vi "generate channels from bitfile registers.vi"(8 "error in":errorcluster, 11 "bitfilefile path":path) -> (0 "error out":errorcluster, 2 "not supported channels":refnum<class "TBM channel.lvclass">[](array[class]), 3 "channels":refnum<class "TBM channel.lvclass">[](array[class]))   [LabVIEW 2014, in "io configuration.lvclass"]
uses:
  io configuration.lvclass
  <vilib>/NI/Tag Bus Module Framework/channel/channel classification.ctl
  <vilib>/NI/Tag Bus Module Framework/channel/TBM channel.lvclass
  <vilib>/NI/Tag Bus/tag/Data Type.ctl
  <vilib>/NI/Tag Bus/tag/tag descriptor.lvclass
  <vilib>/Utility/VariantDataType/VariantType.lvlib
  source/fpga channel/fpga channel.lvclass
  <vilib>/rvi/ClientSDK/Host Interface/DMA/public/niFpgaDmaChannelVisibilityFilter.ctl
  <vilib>/rvi/ClientSDK/Core/ModuleGeneration/CommunicationInterfaceUtility/niFpgaDmaChannelImplementation.ctl
  source/fifo channel/fifo channel.lvclass
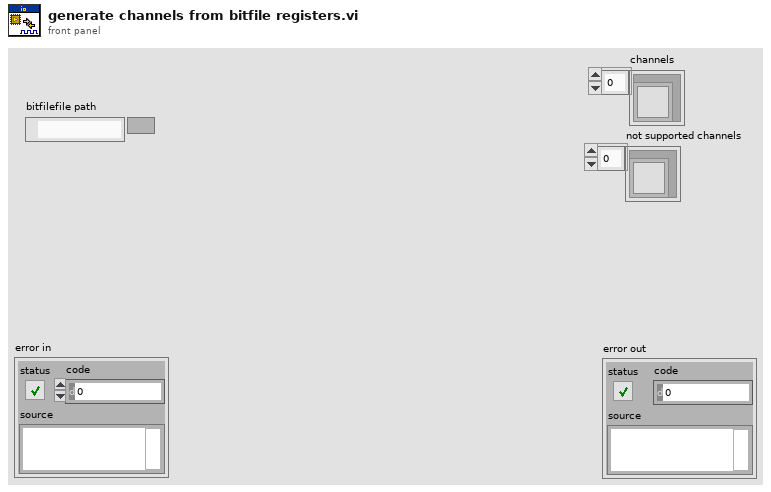
[diagram p1: front panel]
types:
  T1 = typedef "niFpgaDmaChannelVisibilityFilter.ctl" = enum16{"All", "UserVisible"}
  T2 = typedef "nirviReadCallControlInfo.ctl" = cluster{"names":string[], "indicator":bool[], "type descriptor":variant[], "size/rep":u32[], "top level type descriptor":variant[], "level":i32[], "class":string[], "address":i32[], "item orders":cluster{"order":u32[]}[], "name hierarchies":cluster{"name":string[]}[], "access may timeout":bool[], "from register node":bool[]}
  T3 = typedef "Fifo_DMA_Config.ctl" = cluster{"Name":string, "Depth":u32, "Write? (Deprecated:Use Implementation)":bool, "Physical Channel":u32, "Base Address":u32, "Data Width":u32, "Data Type":T4, "FXP Properties":variant, "Write Window Address":u32, "Implementation":T5, "Control Set":u32}
  T4 = typedef "niFpgaDataTypeControl.ctl" = enum32{"Boolean", "I8", "I16", "I32", "I64", "U8", "U16", "U32", "U64", "FXP", "CustomControl", "SGL"}
  T5 = typedef "niFpgaDmaChannelImplementation.ctl" = enum16{"niFpgaTargetToHost", "niFpgaHostToTarget", "niFpgaPeerToPeerWriter", "niFpgaPeerToPeerReader", "niCoreTargetToHost", "niCoreHostToTarget"}
  T6 = typedef "tag bus.lvlib/tag descriptor.lvclass/Data Type.ctl" = enum16{"Double", "Single", "I64", "I32", "I16", "I8", "U64", "U32", "U16", "U8", "Boolean", "String", "Array of Double", "Array of Single", "Array of I64", "Array of I32", "Array of I16", "Array of I8", "Array of U64", "Array of U32", "Array of U16", "Array of U8", "Array of Boolean", "Array of String"}
  T7 = typedef "TBM channel.lvclass/channel classification.ctl" = enum16{"input data", "output data", "processing parameter", "processing result"}
  T8 = typedef "LVFixedPointRepBitsTypeDef.ctl" = cluster{"Signed":bool, "Word Length":u32, "Integer Word Length":i32}
  T9 = typedef "VariantType.lvlib/Type.ctl" = enum8{"Invalid Type", "Void", "I8", "I16", "I32", "I64", "U8", "U16", "U32", "U64", "Single Float", "Double Float", "Extended Float", "Single Complex", "Double Complex", "Extended Complex", "Enum U8", "Enum U16", "Enum U32", "Enum U64", "Single Float With Unit", "Double Float With Unit", "Extended Float With Unit", "Single Complex with Unit", "Double Complex with Unit", "Extended Complex with Unit", "Boolean", "String", "Path", "Picture", "Tag", "Array", "Cluster", "Variant", "LV Variant", "Waveform", "Timestamp", "Digital Waveform", "Digital Data", "ExpressData", "Refnum", "External Data", "VI", "Poly VI", "LabVIEW Class Instance", "Fixed Point"}
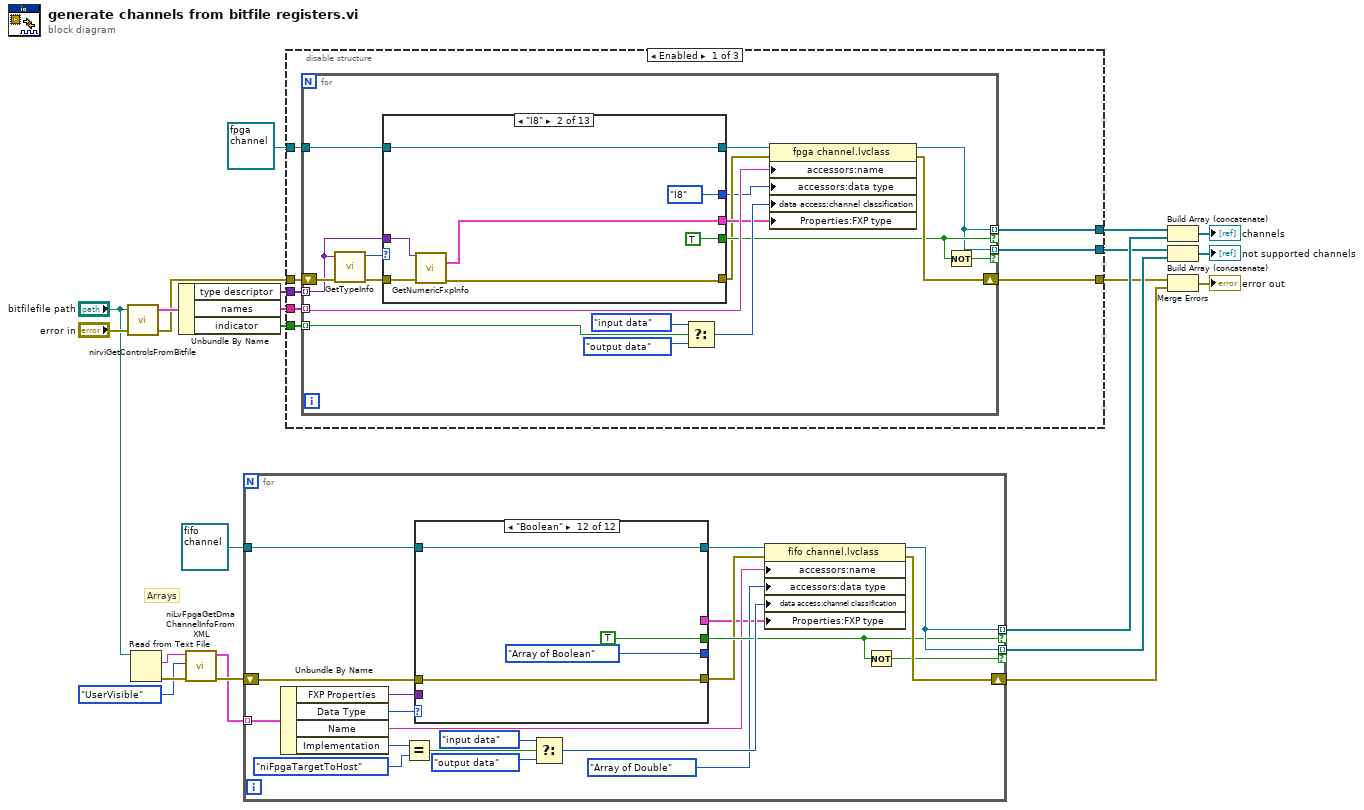
[diagram p0: block diagram]
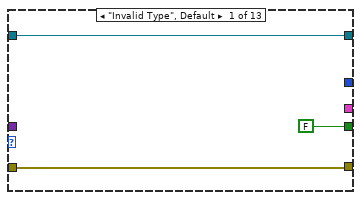
[diagram p2: hidden frame]
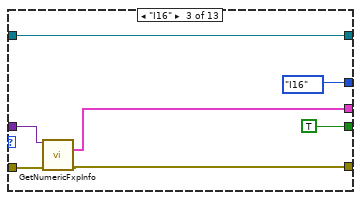
[diagram p3: hidden frame]
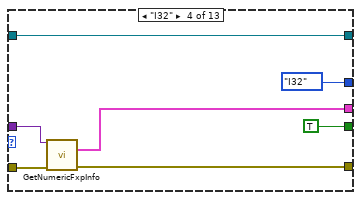
[diagram p4: hidden frame]
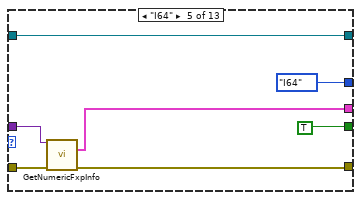
[diagram p5: hidden frame]
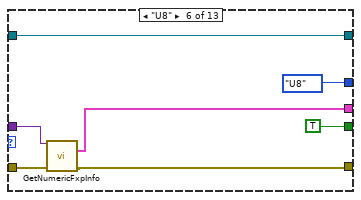
[diagram p6: hidden frame]
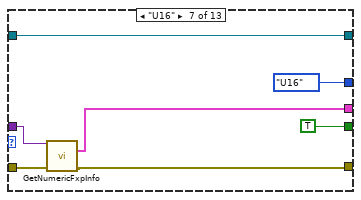
[diagram p7: hidden frame]
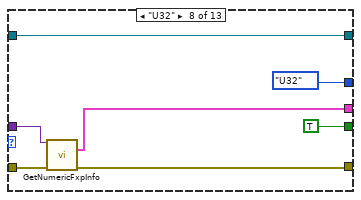
[diagram p8: hidden frame]
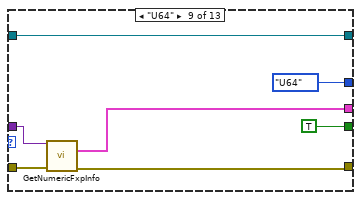
[diagram p9: hidden frame]
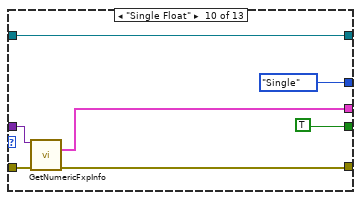
[diagram p10: hidden frame]
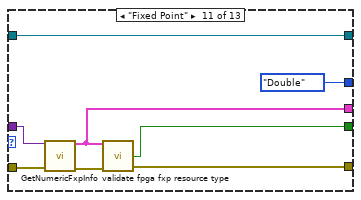
[diagram p11: hidden frame]
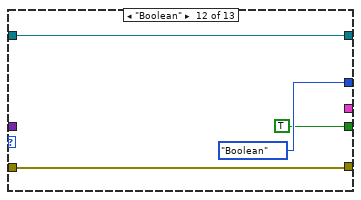
[diagram p12: hidden frame]
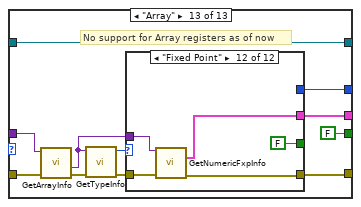
[diagram p13: hidden frame]
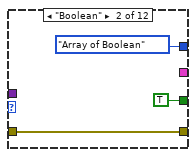
[diagram p15: hidden frame]
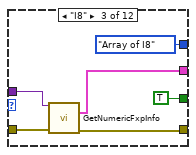
[diagram p16: hidden frame]
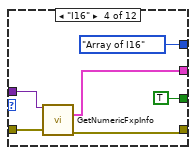
[diagram p17: hidden frame]
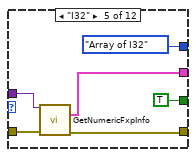
[diagram p18: hidden frame]
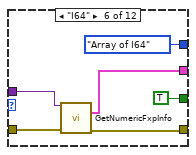
[diagram p19: hidden frame]
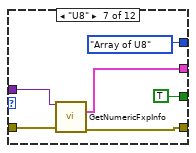
[diagram p20: hidden frame]
diagram:
  # "Arrays"
  n1 = call <vilib>:"nirviGetControlsFromBitfile.vi"("error in (no error)"="error in", "bitfile path"="bitfilefile path") -> ("error out"=w14:errorcluster, "controls"=w15:T2)  [unwired: 2 in]
  n2 = Read from Text File(file (use dialog)="bitfilefile path") -> (text=w19:string, error out=w18:errorcluster)  [unwired: 1 in, 4 out]
  n3 = Unbundle By Name(w15) -> ("type descriptor"=w20:variant[], "names"=w21:string[], "indicator"=w22:bool[])
  n4 = call <resource>:"niLvFpgaGetDmaChannelInfoFromXML.vi"("error in (no error)"=w18, "DMA Channel Filter"=niFpgaDmaChannelVisibilityFilter."UserVisible", "XML String in"=w19) -> ("error out"=w13:errorcluster, "DMA configuration array"=w12:T3[])  [unwired: 7 in]
  n5 = for {
    tunnel: [w38] -> w10 mode=indexing if=w36
    shift-right: [w43] -> w3
    shift-left: w13 -> [w30]
    tunnel: [w38] -> w6 mode=indexing if=w37
    tunnel: w12 -> [w35] mode=indexing
    tunnel: refnum<class "fifo channel.lvclass"> refnum ("fifo channel.lvclass") -> [w24]
    n6 = Unbundle By Name(w35) -> ("FXP Properties"=w28:variant, "Data Type"=w29:T4, "Name"=w34:string, "Implementation"=w33:T5)
    n7 = Equal?(x=w33, y=niFpgaDmaChannelImplementation."niFpgaTargetToHost") -> (x = y?=w31:bool)
    n8 = case shown="\"Boolean\"" w29 {
      tunnel: w30 -> [w45 w50 w57 w64 w71 w78 w85 w92 w99 w106 w117 w119]
      tunnel: [FALSE TRUE TRUE TRUE TRUE TRUE TRUE TRUE TRUE TRUE w114 TRUE] -> w36
      tunnel: [_ Data_Type."Array of I8" ("data type") Data_Type."Array of I16" ("data type") Data_Type."Array of I32" ("data type") Data_Type."Array of I64" ("data type") Data_Type."Array of U8" ("data type") Data_Type."Array of U16" ("data type") Data_Type."Array of U32" ("data type") Data_Type."Array of U64" ("data type") Data_Type."Array of Single" ("data type") Data_Type."Array of Double" ("data type") Data_Type."Array of Boolean" ("data type")] -> _
      tunnel: [w45 w49 w56 w63 w70 w77 w84 w91 w98 w105 w110 w119] -> w26
      tunnel: w24 -> [w44 w51 w58 w65 w72 w79 w86 w93 w100 w107 w112 w118]
      tunnel: [w44 w51 w58 w65 w72 w79 w86 w93 w100 w107 w112 w118] -> w40
      tunnel: w28 -> [_ w47 w54 w61 w68 w75 w82 w89 w96 w103 w113 _]
      tunnel: [_ w48 w55 w62 w69 w76 w83 w90 w97 w104 w111 _] -> w25
      frame Default {
      }
      frame "I8" {
        n9 = call <vilib>:"GetNumericFxpInfo.vi"("Variant"=w47, "error in (no error)"=w50) -> ("FxpRepresentation"=w48:T8, "error out"=w49:errorcluster)  [unwired: 9 in, 3 out]
      }
      frame "I16" {
        n10 = call <vilib>:"GetNumericFxpInfo.vi"("Variant"=w54, "error in (no error)"=w57) -> ("FxpRepresentation"=w55:T8, "error out"=w56:errorcluster)  [unwired: 9 in, 3 out]
      }
      frame "I32" {
        n11 = call <vilib>:"GetNumericFxpInfo.vi"("Variant"=w61, "error in (no error)"=w64) -> ("FxpRepresentation"=w62:T8, "error out"=w63:errorcluster)  [unwired: 9 in, 3 out]
      }
      frame "I64" {
        n12 = call <vilib>:"GetNumericFxpInfo.vi"("Variant"=w68, "error in (no error)"=w71) -> ("FxpRepresentation"=w69:T8, "error out"=w70:errorcluster)  [unwired: 9 in, 3 out]
      }
      frame "U8" {
        n13 = call <vilib>:"GetNumericFxpInfo.vi"("Variant"=w75, "error in (no error)"=w78) -> ("FxpRepresentation"=w76:T8, "error out"=w77:errorcluster)  [unwired: 9 in, 3 out]
      }
      frame "U16" {
        n14 = call <vilib>:"GetNumericFxpInfo.vi"("Variant"=w82, "error in (no error)"=w85) -> ("FxpRepresentation"=w83:T8, "error out"=w84:errorcluster)  [unwired: 9 in, 3 out]
      }
      frame "U32" {
        n15 = call <vilib>:"GetNumericFxpInfo.vi"("Variant"=w89, "error in (no error)"=w92) -> ("FxpRepresentation"=w90:T8, "error out"=w91:errorcluster)  [unwired: 9 in, 3 out]
      }
      frame "U64" {
        n16 = call <vilib>:"GetNumericFxpInfo.vi"("Variant"=w96, "error in (no error)"=w99) -> ("FxpRepresentation"=w97:T8, "error out"=w98:errorcluster)  [unwired: 9 in, 3 out]
      }
      frame "SGL" {
        n17 = call <vilib>:"GetNumericFxpInfo.vi"("Variant"=w103, "error in (no error)"=w106) -> ("FxpRepresentation"=w104:T8, "error out"=w105:errorcluster)  [unwired: 9 in, 3 out]
      }
      frame "FXP" {
        n18 = call <vilib>:"GetNumericFxpInfo.vi"("Variant"=w113, "error in (no error)"=w117) -> ("FxpRepresentation"=w111:T8, "error out"=w116:errorcluster)  [unwired: 9 in, 3 out]
        n19 = call "validate fpga fxp resource type.vi"("FXP Representation"=w111, "error in (no error)"=w116) -> ("FXP type supported"=w114:bool, "error out"=w110:errorcluster)  [unwired: 11 in, 1 out]
      }
      frame "Boolean" {
      }
    }
    n20 = Select(t=channel_classification."input data" ("channel classification"), s=w31, f=channel_classification."output data" ("channel classification")) -> (s? t:f=w39:T7)
    n21 = property class="fifo channel.lvclass"(reference=w40, error in=w26, "accessors:name"=w34, "accessors:data type"=Data_Type."Array of Double" ("data type"), "data access:channel classification"=w39, "Properties:FXP type"=w25) -> (reference out=w38:refnum<class "fifo channel.lvclass">, error out=w43:errorcluster)
    n22 = Not(x=w36) -> (.not. x?=w37:bool)
  }
  n23 = disable-structure shown="Enabled" {
    disable-tunnel: w22 -> [w129 w306 w406]
    disable-tunnel: w21 -> [w128 w305 w405]
    disable-tunnel: w20 -> [w127 w304 w404]
    disable-tunnel: w14 -> [w126 w303 w403]
    disable-tunnel: [w125 w302 w402] -> w11
    disable-tunnel: [w124 w301 w401] -> w7
    disable-tunnel: [w123 w300 w400] -> w4
    disable-tunnel: refnum<class "fpga channel.lvclass"> refnum ("Fxp Channel.lvclass") -> [w122 w299 _]
    frame Enabled {
      n24 = for {
        tunnel: [w132] -> w125 mode=indexing if=w133
        tunnel: w129 -> [w142] mode=indexing
        tunnel: w128 -> [w140] mode=indexing
        tunnel: w127 -> [w135] mode=indexing
        shift-right: [w147] -> w123
        shift-left: w126 -> [w146]
        tunnel: [w132] -> w124 mode=indexing if=w138
        tunnel: w122 -> [w137]
        n25 = call <vilib>:"GetTypeInfo.vi"("error in (no error)"=w146, "Variant"=w135) -> ("error out"=w143:errorcluster, "Type Enum"=w136:T9)  [unwired: 5 in, 3 out]
        n26 = case shown="\"I8\"" w136 {
          tunnel: w143 -> [w149 w154 w161 w168 w175 w182 w189 w196 w203 w210 w219 w223 w234]
          tunnel: [FALSE TRUE TRUE TRUE TRUE TRUE TRUE TRUE TRUE TRUE w214 TRUE FALSE ("FXP type supported")] -> w133
          tunnel: [_ Data_Type."I8" ("data type") Data_Type."I16" ("data type") Data_Type."I32" ("data type") Data_Type."I64" ("data type") Data_Type."U8" ("data type") Data_Type."U16" ("data type") Data_Type."U32" ("data type") Data_Type."U64" ("data type") Data_Type."Single" ("data type") Data_Type."Double" ("data type") Data_Type."Boolean" ("data type") w231] -> w130
          tunnel: [w149 w153 w160 w165 w173 w181 w188 w195 w202 w208 w215 w223 w227] -> w131
          tunnel: w137 -> [w148 w155 w162 w169 w176 w183 w190 w197 w204 w211 w220 w222 w233]
          tunnel: [w148 w155 w162 w169 w176 w183 w190 w197 w204 w211 w220 w222 w233] -> w141
          tunnel: w135 -> [_ w152 w159 w167 w174 w180 w187 w194 w201 w209 w218 _ w232]
          tunnel: [_ w151 w158 w166 w172 w179 w186 w193 w200 w207 w216 _ w226] -> w134
          frame "Invalid Type", Default {
          }
          frame "I8" {
            n27 = call <vilib>:"GetNumericFxpInfo.vi"("Variant"=w152, "error in (no error)"=w154) -> ("FxpRepresentation"=w151:T8, "error out"=w153:errorcluster)  [unwired: 9 in, 3 out]
          }
          frame "I16" {
            n28 = call <vilib>:"GetNumericFxpInfo.vi"("Variant"=w159, "error in (no error)"=w161) -> ("FxpRepresentation"=w158:T8, "error out"=w160:errorcluster)  [unwired: 9 in, 3 out]
          }
          frame "I32" {
            n29 = call <vilib>:"GetNumericFxpInfo.vi"("Variant"=w167, "error in (no error)"=w168) -> ("FxpRepresentation"=w166:T8, "error out"=w165:errorcluster)  [unwired: 9 in, 3 out]
          }
          frame "I64" {
            n30 = call <vilib>:"GetNumericFxpInfo.vi"("Variant"=w174, "error in (no error)"=w175) -> ("FxpRepresentation"=w172:T8, "error out"=w173:errorcluster)  [unwired: 9 in, 3 out]
          }
          frame "U8" {
            n31 = call <vilib>:"GetNumericFxpInfo.vi"("Variant"=w180, "error in (no error)"=w182) -> ("FxpRepresentation"=w179:T8, "error out"=w181:errorcluster)  [unwired: 9 in, 3 out]
          }
          frame "U16" {
            n32 = call <vilib>:"GetNumericFxpInfo.vi"("Variant"=w187, "error in (no error)"=w189) -> ("FxpRepresentation"=w186:T8, "error out"=w188:errorcluster)  [unwired: 9 in, 3 out]
          }
          frame "U32" {
            n33 = call <vilib>:"GetNumericFxpInfo.vi"("Variant"=w194, "error in (no error)"=w196) -> ("FxpRepresentation"=w193:T8, "error out"=w195:errorcluster)  [unwired: 9 in, 3 out]
          }
          frame "U64" {
            n34 = call <vilib>:"GetNumericFxpInfo.vi"("Variant"=w201, "error in (no error)"=w203) -> ("FxpRepresentation"=w200:T8, "error out"=w202:errorcluster)  [unwired: 9 in, 3 out]
          }
          frame "Single Float" {
            n35 = call <vilib>:"GetNumericFxpInfo.vi"("Variant"=w209, "error in (no error)"=w210) -> ("FxpRepresentation"=w207:T8, "error out"=w208:errorcluster)  [unwired: 9 in, 3 out]
          }
          frame "Fixed Point" {
            n36 = call <vilib>:"GetNumericFxpInfo.vi"("Variant"=w218, "error in (no error)"=w219) -> ("FxpRepresentation"=w216:T8, "error out"=w217:errorcluster)  [unwired: 9 in, 3 out]
            n37 = call "validate fpga fxp resource type.vi"("FXP Representation"=w216, "error in (no error)"=w217) -> ("FXP type supported"=w214:bool, "error out"=w215:errorcluster)  [unwired: 11 in, 1 out]
          }
          frame "Boolean" {
          }
          frame "Array" {
            # "No support for Array registers as of now"
            n38 = call <vilib>:"GetArrayInfo.vi"("error in (no error)"=w234, "Variant"=w232) -> ("error out"=w235:errorcluster, "ArrayElement"=w229:variant)  [unwired: 6 in, 2 out]
            n39 = call <vilib>:"GetTypeInfo.vi"("error in (no error)"=w235, "Variant"=w229) -> ("error out"=w228:errorcluster, "Type Enum"=w236:T9)  [unwired: 5 in, 3 out]
            n40 = case shown="\"Fixed Point\"" w236 {
              tunnel: [_ Data_Type."Array of Boolean" ("data type") Data_Type."Array of I8" ("data type") Data_Type."Array of I16" ("data type") Data_Type."Array of I32" ("data type") Data_Type."Array of I64" ("data type") Data_Type."Array of U8" ("data type") Data_Type."Array of U16" ("data type") Data_Type."Array of U32" ("data type") Data_Type."Array of U64" ("data type") Data_Type."Array of Single" ("data type") _] -> w231
              tunnel: [_ TRUE TRUE TRUE TRUE TRUE TRUE TRUE TRUE TRUE TRUE FALSE] -> _
              tunnel: w229 -> [_ _ w243 w249 w255 w261 w267 w273 w278 w285 w290 w296]
              tunnel: w228 -> [w237 w238 w244 w250 w256 w262 w268 w274 w279 w284 w291 w297]
              tunnel: [w237 w238 w242 w248 w254 w260 w266 w272 w277 w283 w289 w294] -> w227
              tunnel: [_ _ w241 w247 w253 w259 w265 w271 _ w282 w288 w295] -> w226
              frame "Invalid Type", Default {
              }
              frame "Boolean" {
              }
              frame "I8" {
                n41 = call <vilib>:"GetNumericFxpInfo.vi"("Variant"=w243, "error in (no error)"=w244) -> ("FxpRepresentation"=w241:T8, "error out"=w242:errorcluster)  [unwired: 9 in, 3 out]
              }
              frame "I16" {
                n42 = call <vilib>:"GetNumericFxpInfo.vi"("Variant"=w249, "error in (no error)"=w250) -> ("FxpRepresentation"=w247:T8, "error out"=w248:errorcluster)  [unwired: 9 in, 3 out]
              }
              frame "I32" {
                n43 = call <vilib>:"GetNumericFxpInfo.vi"("Variant"=w255, "error in (no error)"=w256) -> ("FxpRepresentation"=w253:T8, "error out"=w254:errorcluster)  [unwired: 9 in, 3 out]
              }
              frame "I64" {
                n44 = call <vilib>:"GetNumericFxpInfo.vi"("Variant"=w261, "error in (no error)"=w262) -> ("FxpRepresentation"=w259:T8, "error out"=w260:errorcluster)  [unwired: 9 in, 3 out]
              }
              frame "U8" {
                n45 = call <vilib>:"GetNumericFxpInfo.vi"("Variant"=w267, "error in (no error)"=w268) -> ("FxpRepresentation"=w265:T8, "error out"=w266:errorcluster)  [unwired: 9 in, 3 out]
              }
              frame "U16" {
                n46 = call <vilib>:"GetNumericFxpInfo.vi"("Variant"=w273, "error in (no error)"=w274) -> ("FxpRepresentation"=w271:T8, "error out"=w272:errorcluster)  [unwired: 9 in, 3 out]
              }
              frame "U32" {
                n47 = call <vilib>:"GetNumericFxpInfo.vi"("Variant"=w278, "error in (no error)"=w279) -> ("error out"=w277:errorcluster)  [unwired: 9 in, 4 out]
              }
              frame "U64" {
                n48 = call <vilib>:"GetNumericFxpInfo.vi"("Variant"=w285, "error in (no error)"=w284) -> ("FxpRepresentation"=w282:T8, "error out"=w283:errorcluster)  [unwired: 9 in, 3 out]
              }
              frame "Single Float" {
                n49 = call <vilib>:"GetNumericFxpInfo.vi"("Variant"=w290, "error in (no error)"=w291) -> ("FxpRepresentation"=w288:T8, "error out"=w289:errorcluster)  [unwired: 9 in, 3 out]
              }
              frame "Fixed Point" {
                n50 = call <vilib>:"GetNumericFxpInfo.vi"("Variant"=w296, "error in (no error)"=w297) -> ("FxpRepresentation"=w295:T8, "error out"=w294:errorcluster)  [unwired: 9 in, 3 out]
              }
            }
          }
        }
        n51 = Select(t=channel_classification."input data" ("channel classification"), s=w142, f=channel_classification."output data" ("channel classification")) -> (s? t:f=w139:T7)
        n52 = property class="fpga channel.lvclass"(reference=w141, error in=w131, "accessors:name"=w140, "accessors:data type"=w130, "data access:channel classification"=w139, "Properties:FXP type"=w134) -> (reference out=w132:refnum<class "fpga channel.lvclass">, error out=w147:errorcluster)
        n53 = Not(x=w133) -> (.not. x?=w138:bool)
      }
    }
    frame Disabled {
      n54 = for {
        tunnel: [w313] -> w302 mode=indexing if=w307
        tunnel: w306 -> [w320] mode=indexing
        tunnel: w305 -> [w318] mode=indexing
        tunnel: w304 -> [w311] mode=indexing
        shift-right: [w312] -> w300
        shift-left: w303 -> [w324]
        tunnel: [w313] -> w301 mode=indexing if=w315
        tunnel: w299 -> [w310]
        n55 = call <vilib>:"GetTypeInfo.vi"("error in (no error)"=w324, "Variant"=w311) -> ("error out"=w321:errorcluster, "Type Enum"=w309:T9)  [unwired: 5 in, 3 out]
        n56 = case shown="\"I8\"" w309 {
          tunnel: w321 -> [w326 w329 w333 w337 w341 w345 w349 w353 w357 w361 w365 w369 w374]
          tunnel: w311 -> [_ _ _ _ _ _ _ _ _ _ _ _ w373]
          tunnel: [FALSE TRUE TRUE TRUE TRUE TRUE TRUE TRUE TRUE TRUE TRUE TRUE _] -> w308
          tunnel: [_ Data_Type."I8" ("data type") Data_Type."I16" ("data type") Data_Type."I32" ("data type") Data_Type."I64" ("data type") Data_Type."U8" ("data type") Data_Type."U16" ("data type") Data_Type."U32" ("data type") Data_Type."U64" ("data type") Data_Type."Single" ("data type") Data_Type."Double" ("data type") Data_Type."Boolean" ("data type") _] -> w317
          tunnel: [w326 w329 w333 w337 w341 w345 w349 w353 w357 w361 w365 w369 w378] -> w312
          tunnel: w310 -> [w325 w328 w332 w336 w340 w344 w348 w352 w356 w360 w366 w368 w372]
          tunnel: [w325 w328 w332 w336 w340 w344 w348 w352 w356 w360 w366 w368 w372] -> w319
          frame "Invalid Type", Default {
          }
          frame "I8" {
          }
          frame "I16" {
          }
          frame "I32" {
          }
          frame "I64" {
          }
          frame "U8" {
          }
          frame "U16" {
          }
          frame "U32" {
          }
          frame "U64" {
          }
          frame "Single Float" {
          }
          frame "Fixed Point" {
          }
          frame "Boolean" {
          }
          frame "Array" {
            # "No support for Array registers as of now"
            n57 = call <vilib>:"GetArrayInfo.vi"("error in (no error)"=w374, "Variant"=w373) -> ("error out"=w376:errorcluster, "ArrayElement"=w375:variant)  [unwired: 6 in, 2 out]
            n58 = call <vilib>:"GetTypeInfo.vi"("error in (no error)"=w376, "Variant"=w375) -> ("error out"=w378:errorcluster, "Type Enum"=w377:T9)  [unwired: 5 in, 3 out]
            n59 = case shown="\"U32\"" w377 {
              tunnel: [_ Data_Type."Array of Boolean" ("data type") Data_Type."Array of I8" ("data type") Data_Type."Array of I16" ("data type") Data_Type."Array of I32" ("data type") Data_Type."Array of I64" ("data type") Data_Type."Array of U8" ("data type") Data_Type."Array of U16" ("data type") Data_Type."Array of U32" ("data type") Data_Type."Array of U64" ("data type") Data_Type."Array of Single" ("data type") _] -> _
              tunnel: [_ TRUE TRUE TRUE TRUE TRUE TRUE TRUE TRUE TRUE TRUE FALSE] -> _
              frame "Invalid Type", Default {
              }
              frame "Boolean" {
              }
              frame "I8" {
              }
              frame "I16" {
              }
              frame "I32" {
              }
              frame "I64" {
              }
              frame "U8" {
              }
              frame "U16" {
              }
              frame "U32" {
              }
              frame "U64" {
              }
              frame "Single Float" {
              }
              frame "Fixed Point" {
              }
            }
          }
        }
        n60 = Select(t=channel_classification."input data" ("channel classification"), s=w320, f=channel_classification."output data" ("channel classification")) -> (s? t:f=w316:T7)
        n61 = property class="fpga channel.lvclass"(reference=w319, "accessors:name"=w318, "accessors:data type"=w317, "data access:channel classification"=w316) -> (reference out=w314:refnum<class "fpga channel.lvclass">)  [unwired: 1 in, 1 out]
        n62 = Not() -> (x=w307:bool, .not. x?=w315:bool)
      }
    }
    frame Disabled {
      n63 = for {
        tunnel: [w412] -> w402 mode=indexing if=w409
        tunnel: w406 -> [w418] mode=indexing
        tunnel: w405 -> [w416] mode=indexing
        tunnel: w404 -> [w411] mode=indexing
        shift-right: [w413] -> w400
        shift-left: w403 -> [w422]
        tunnel: [w412] -> w401 mode=indexing if=w410
        n64 = call <vilib>:"GetTypeInfo.vi"("error in (no error)"=w422, "Variant"=w411) -> ("error out"=w419:errorcluster, "Type Enum"=w408:T9)  [unwired: 5 in, 3 out]
        n65 = case shown="\"Fixed Point\"" w408 {
          tunnel: w419 -> [w424 w427 w431 w435 w439 w443 w447 w451 w455 w459 w470 w473 w478]
          tunnel: w411 -> [_ _ _ _ _ _ _ _ _ _ _ _ w477]
          tunnel: [FALSE TRUE TRUE TRUE TRUE TRUE TRUE TRUE TRUE TRUE w464 TRUE w483] -> w409
          tunnel: [_ Data_Type."I8" ("data type") Data_Type."I16" ("data type") Data_Type."I32" ("data type") Data_Type."I64" ("data type") Data_Type."U8" ("data type") Data_Type."U16" ("data type") Data_Type."U32" ("data type") Data_Type."U64" ("data type") Data_Type."Single" ("data type") Data_Type."Double" ("data type") Data_Type."Boolean" ("data type") w484] -> w415
          tunnel: [w424 w427 w431 w435 w439 w443 w447 w451 w455 w459 w468 w473 w482] -> w413
          tunnel: w411 -> [_ _ _ _ _ _ _ _ _ _ w471 _ _]
          tunnel: refnum<class "fpga channel.lvclass"> refnum ("Fxp Channel.lvclass") -> [w423 w426 w430 w434 w438 w442 w446 w450 w454 w458 w462 w472 w476]
          tunnel: [w423 w426 w430 w434 w438 w442 w446 w450 w454 w458 w469 w472 w476] -> w417
          frame "Invalid Type", Default {
          }
          frame "I8" {
          }
          frame "I16" {
          }
          frame "I32" {
          }
          frame "I64" {
          }
          frame "U8" {
          }
          frame "U16" {
          }
          frame "U32" {
          }
          frame "U64" {
          }
          frame "Single Float" {
          }
          frame "Fixed Point" {
            n66 = call <vilib>:"GetNumericFxpInfo.vi"("error in (no error)"=w470, "Variant"=w471) -> ("error out"=w467:errorcluster, "FXP Representation"=w463:T8)  [unwired: 6 in, 2 out]
            n67 = call "validate fpga fxp resource type.vi"("FXP Representation"=w463, "error in (no error)"=w467) -> ("FXP type supported"=w464:bool, "error out"=w466:errorcluster)  [unwired: 11 in, 1 out]
            n68 = property class="fpga channel.lvclass"(reference=w462, error in=w466, "Properties:FXP type"=w463) -> (reference out=w469:refnum<class "fpga channel.lvclass">, error out=w468:errorcluster)
          }
          frame "Boolean" {
          }
          frame "Array" {
            n69 = call <vilib>:"GetArrayInfo.vi"("error in (no error)"=w478, "Variant"=w477) -> ("error out"=w480:errorcluster, "ArrayElement"=w479:variant)  [unwired: 6 in, 2 out]
            n70 = call <vilib>:"GetTypeInfo.vi"("error in (no error)"=w480, "Variant"=w479) -> ("error out"=w482:errorcluster, "Type Enum"=w481:T9)  [unwired: 5 in, 3 out]
            n71 = case shown="\"Invalid Type\", Default" w481 {
              tunnel: [_ Data_Type."Array of Boolean" ("data type") Data_Type."Array of I8" ("data type") Data_Type."Array of I16" ("data type") Data_Type."Array of I32" ("data type") Data_Type."Array of I64" ("data type") Data_Type."Array of U8" ("data type") Data_Type."Array of U16" ("data type") Data_Type."Array of U32" ("data type") Data_Type."Array of U64" ("data type") Data_Type."Array of Single" ("data type") _] -> w484
              tunnel: [_ TRUE TRUE TRUE TRUE TRUE TRUE TRUE TRUE TRUE TRUE FALSE] -> w483
              frame "Invalid Type", Default {
              }
              frame "Boolean" {
              }
              frame "I8" {
              }
              frame "I16" {
              }
              frame "I32" {
              }
              frame "I64" {
              }
              frame "U8" {
              }
              frame "U16" {
              }
              frame "U32" {
              }
              frame "U64" {
              }
              frame "Single Float" {
              }
              frame "Fixed Point" {
              }
            }
          }
        }
        n72 = Select(t=channel_classification."input data" ("channel classification"), s=w418, f=channel_classification."output data" ("channel classification")) -> (s? t:f=w414:T7)
        n73 = property class="fpga channel.lvclass"(reference=w417, "accessors:name"=w416, "accessors:data type"=w415, "data access:channel classification"=w414) -> (reference out=w412:refnum<class "fpga channel.lvclass">)  [unwired: 1 in, 1 out]
        n74 = Not(x=w409) -> (.not. x?=w410:bool)
      }
    }
  }
  n75 = Build Array (concatenate)(w11, w10) -> (→"channels":refnum<class "TBM channel.lvclass">[])
  n76 = Build Array (concatenate)(w7, w6) -> (→"not supported channels":refnum<class "TBM channel.lvclass">[])
  n77 = Merge Errors(w4, w3) -> (→"error out":errorcluster)
